vi "BarCode.vi"(7 "BC DIGIT":i32) -> (0 "Project Model":string, 1 "Match":bool, 2 "Ok STS":bool, 3 "BarCode_Out":string, 4 "BarCode Exit":bool)   [LabVIEW 2018]
panel:
  out "Boolean":bool
  in  "OK":bool
  out "Status":bool
  in  "stop":bool
  in  "CLEAR":bool
  in  "BarCode":string
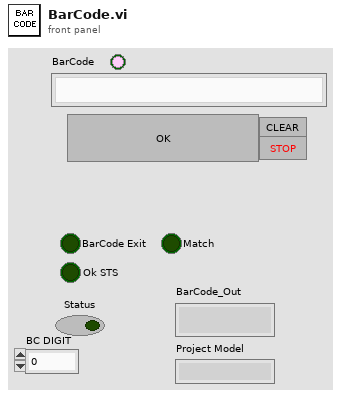
[diagram p1: front panel]
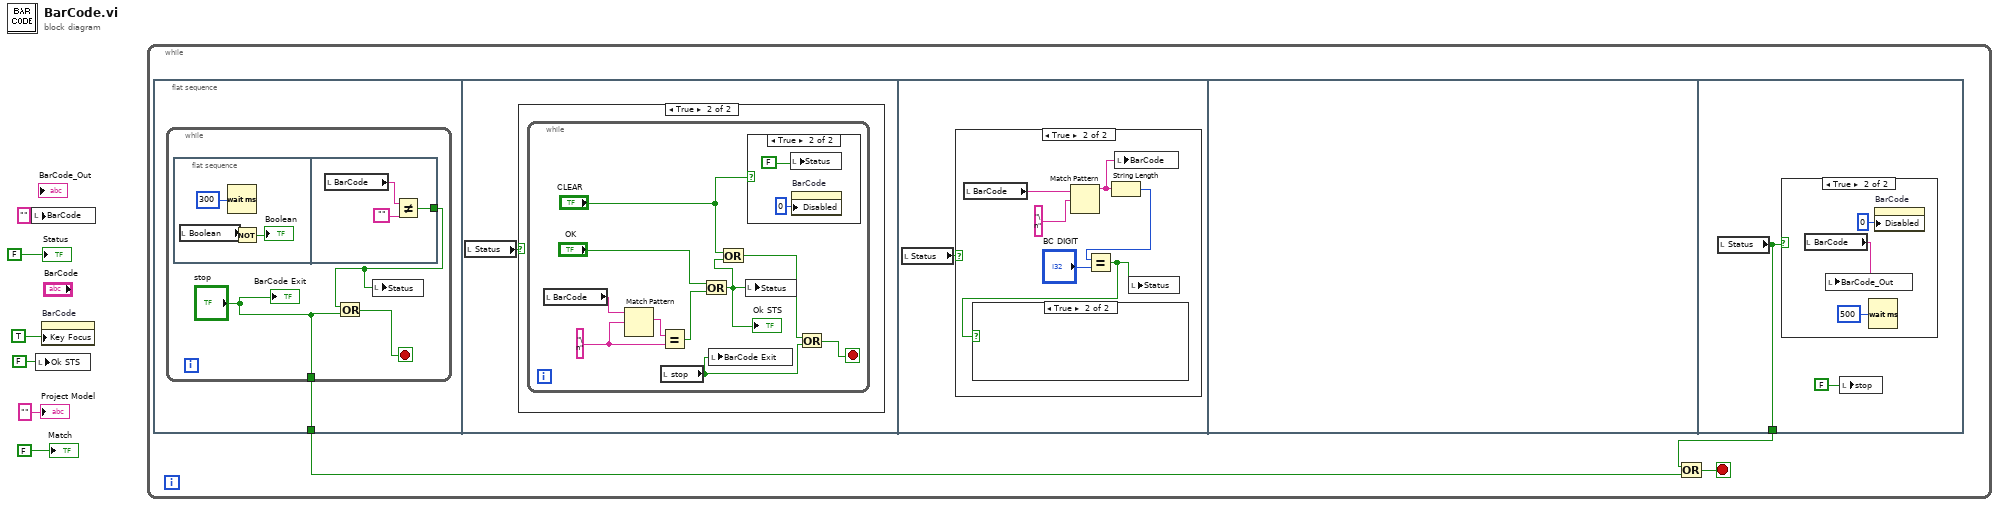
[diagram p0: block diagram]
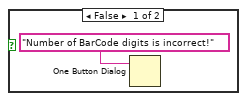
[diagram p5: hidden frame]
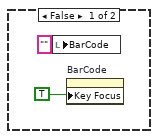
[diagram p6: hidden frame]
diagram:
  n1 = local write "BarCode"("" ("BarCode")) -> ()
  n2 = local write "Ok STS"(FALSE ("OutOk")) -> ()
  n3 = property on="BarCode" class="Str"("Key Focus"=TRUE) -> ()  [unwired: 2 in, 2 out]
  n4 = while {
    stop <- w9 stop-if-true
    n5 = flat-sequence {
      tunnel: [w10] -> w7
      tunnel: [w42] -> w8
      frame #0 {
        n6 = while {
          tunnel: ["stop"] -> w10
          stop <- w12 stop-if-true
          n7 = flat-sequence {
            tunnel: [w17] -> w13
            frame #0 {
              n8 = local read "Boolean"() -> (w14:bool)
              n9 = Wait (ms)(milliseconds to wait=u32 300) -> ()  [unwired: 1 out]
              n10 = Not(x=w14) -> (.not. x?=→"Boolean":bool)
            }
            frame #1 {
              n11 = local read "BarCode"() -> (w19:string)
              n12 = Not Equal?(x=w19, y="") -> (x != y?=w17:bool)
            }
          }
          n13 = Or(x=w13, y="stop") -> (x .or. y?=w12:bool)
          n14 = local write "Status"(w13) -> ()
          "BarCode Exit" <- "stop"
        }
      }
      frame #1 {
        n15 = local read "Status"() -> (w20:bool)
        n16 = case shown="True" w20 {
          frame False {
          }
          frame True {
            n17 = while {
              stop <- w30 stop-if-true
              w21 = "\n"
              n18 = local read "BarCode"() -> (w26:string)
              n19 = Match Pattern(string=w26, regular expression=w21) -> (match substring=w25:string)  [unwired: 4 out]
              n20 = Equal?(x=w25, y=w21) -> (x = y?=w24:bool)
              n21 = local read "stop"() -> (w29:bool)
              n22 = Or(x="OK", y=w24) -> (x .or. y?=w22:bool)
              "Ok STS" <- w22
              n23 = local write "BarCode Exit"(w29) -> ()
              n24 = Or(x="CLEAR", y=w22) -> (x .or. y?=w27:bool)
              n25 = local write "Status"(w22) -> ()
              n26 = case shown="True" "CLEAR" {
                frame False {
                }
                frame True {
                  n27 = local write "Status"(FALSE ("Status")) -> ()
                  n28 = property on="BarCode" class="Str"("Disabled"=u8 0) -> ()  [unwired: 2 in, 2 out]
                }
              }
              n29 = Or(x=w27, y=w29) -> (x .or. y?=w30:bool)
            }
          }
        }
      }
      frame #2 {
        n30 = local read "Status"() -> (w33:bool)
        n31 = case shown="True" w33 {
          frame False {
          }
          frame True {
            n32 = local read "BarCode"() -> (w38:string)
            n33 = Match Pattern(string=w38, regular expression="\n") -> (before substring=w35:string)  [unwired: 4 out]
            n34 = String Length(string=w35) -> (length=w37:i32)
            n35 = Equal?(x=w37, y="BC DIGIT") -> (x = y?=w36:bool)
            n36 = case shown="True" w36 {
              frame False {
                n37 = One Button Dialog(message="Number of BarCode digits is incorrect!") -> ()  [unwired: 2 out]
              }
              frame True {
              }
            }
            n38 = local write "BarCode"(w35) -> ()
            n39 = local write "Status"(w36) -> ()
          }
        }
      }
      frame #3 {
      }
      frame #4 {
        n40 = local read "Status"() -> (w42:bool)
        n41 = case shown="True" w42 {
          frame False {
            n42 = local write "BarCode"("" ("BarCode")) -> ()
            n43 = property on="BarCode" class="Str"("Key Focus"=TRUE) -> ()  [unwired: 2 in, 2 out]
          }
          frame True {
            n44 = local read "BarCode"() -> (w47:string)
            n45 = local write "BarCode_Out"(w47) -> ()
            n46 = Wait (ms)(milliseconds to wait=u32 500) -> ()  [unwired: 1 out]
            n47 = property on="BarCode" class="Str"("Disabled"=u8 0) -> ()  [unwired: 2 in, 2 out]
          }
        }
        n48 = local write "stop"(FALSE ("stop")) -> ()
      }
    }
    n49 = Or(x=w8, y=w7) -> (x .or. y?=w9:bool)
  }
  "Status" <- FALSE ("Status")
  "Project Model" <- "" ("Project Model")
  "Match" <- FALSE ("Match")
